vi "get_nodes_with_no_predecessors.vi"(11 "DiGraph in":refnum<class "DiGraph.lvclass">) -> (1 "node-ids (no predecessors)":refnum<class "ID.lvclass">[](array[class]))   [LabVIEW 2020, in "graph.lvlib" / "DiGraph.lvclass"]
uses:
  DiGraph.lvclass
  DiGraph.lvclass/DiGraph.ctl
  Graph/Graph.lvclass
  C:/Projects/labview-project-load-tools/source/submodules/graph-api-labview/source/api/Graph/Graph.lvclass
  C:/Projects/labview-project-load-tools/source/submodules/graph-api-labview/source/api/DiGraph/DiGraph.lvclass
  ID/ID.lvclass
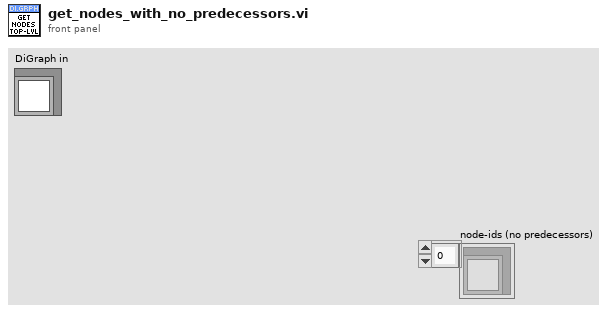
[diagram p1: front panel]
types:
  T1 = map{refnum<class "ID.lvclass">, set{refnum<class "ID.lvclass">}}
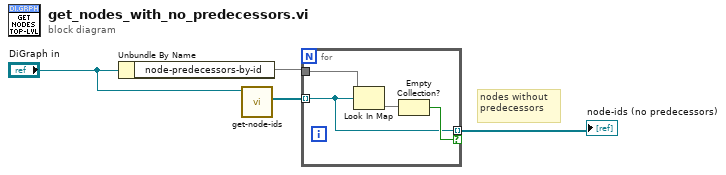
[diagram p0: block diagram]
diagram:
  # "nodes without predecessors"
  n1 = Unbundle By Name("DiGraph in") -> ("node-predecessors-by-id"=w3:T1)
  n2 = call "get-node-ids.vi"("Graph in"="DiGraph in") -> ("node-ids"=w2:refnum<class "ID.lvclass">[])  [unwired: 10 in]
  n3 = for {
    tunnel: w2 -> [w5] mode=indexing
    tunnel: w3 -> [w8]
    tunnel: [w5] -> w4 mode=indexing if=w7
    n4 = Look In Map(map=w8, key=w5) -> (value=w6:set{refnum<class "ID.lvclass">})  [unwired: 1 in, 1 out]
    n5 = Empty Collection?(1:w6) -> (0:w7:bool)
  }
  "node-ids (no predecessors)" <- w4
